vi "Get Scene Window.vi"(0 "Display State In":T1={"Pause"=FALSE, "Camera"={"Position"={"X"=0.0, "Y"=0.0, "Z"=4.0}, "Target"={"X"=0.0, "Y"=0.0, "Z"=0.0}, "Up Direction"={"X"=0.0, "Y"=1.0, "Z"=0.0}}, "Background Color"={"Red"=0.0, "Green"=0.0, "Blue"=0.0, "Alpha"=0.0}, "3DRefnum"=refnum}, 9 "Container State":T3, 11 "error in (no error)":errorcluster) -> (4 "Display State Out":T1={"Pause"=FALSE, "Camera"={"Position"={"X"=0.0, "Y"=0.0, "Z"=4.0}, "Target"={"X"=0.0, "Y"=0.0, "Z"=0.0}, "Up Direction"={"X"=0.0, "Y"=1.0, "Z"=0.0}}, "Background Color"={"Red"=0.0, "Green"=0.0, "Blue"=0.0, "Alpha"=0.0}, "3DRefnum"=refnum}, 6 "SceneWindow":refnum<vi>, 15 "error out":errorcluster)   [LabVIEW 2017, in "Simulator Display.xctl"]
uses:
  <vilib>/robotics/Controls/Simulator Display/Simulator Display.xctl
  <vilib>/_xctls/Container State.ctl
  <vilib>/robotics/Controls/Simulator Display/State.ctl
  <vilib>/Utility/miscctls.llb/LVRGBAColorTypeDef.ctl
  <vilib>/_xctls/XControlSupport.lvlib
panel:
  # "Add Controls & Indicators that form the parameters of the method here. Hook them to the connector pane. Do not delete the controls & indicators that are already hooked to the connector pane.\n \nTo setup the parameters  for this method, right click on this item in the Project Tree & select \"Configure Method...\"."
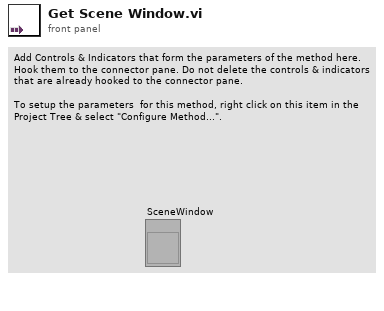
[diagram p1: front panel]
types:
  T1 = typedef "Simulator Display.xctl/State.ctl" = cluster{"Pause":bool, "Camera":cluster{"Position":cluster{"X":dbl, "Y":dbl, "Z":dbl}, "Target":cluster{"X":dbl, "Y":dbl, "Z":dbl}, "Up Direction":cluster{"X":dbl, "Y":dbl, "Z":dbl}}, "Background Color":T2, "3DRefnum":refnum<vi>}
  T2 = typedef "LVRGBAColorTypeDef.ctl" = cluster{"Red":sgl, "Green":sgl, "Blue":sgl, "Alpha":sgl}
  T3 = typedef "XControlSupport.lvlib/Container State.ctl" = cluster{"Indicator?":bool, "Run Mode?":bool, " Refnum":refnum<vi>}
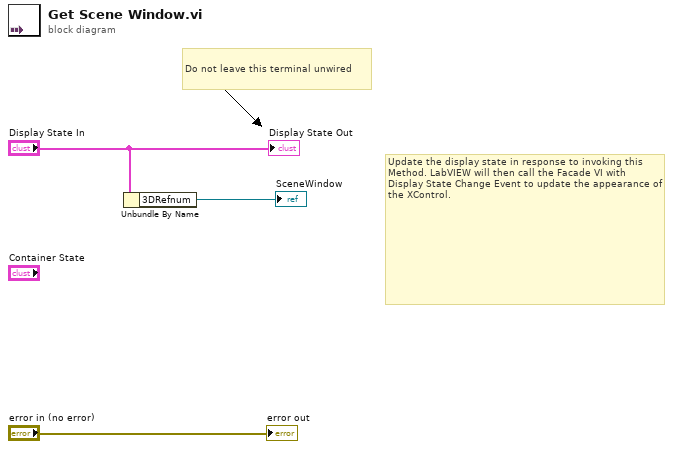
[diagram p0: block diagram]
diagram:
  # "Do not leave this terminal unwired"
  # "Update the display state in response to invoking this Method. LabVIEW will then call the Facade VI with Display State Change Event to update the appearance of the XControl."
  n1 = Unbundle By Name("Display State In") -> ("3DRefnum"=→"SceneWindow":refnum<vi>)
  "Display State Out" <- "Display State In"
  "error out" <- "error in (no error)"
